vi "Read_From_File.vi"(8 "error in":errorcluster, 11 "user":i32) -> (0 "error out":errorcluster, 3 "Events":string)   [LabVIEW 2019]
panel:
  out "user":i32
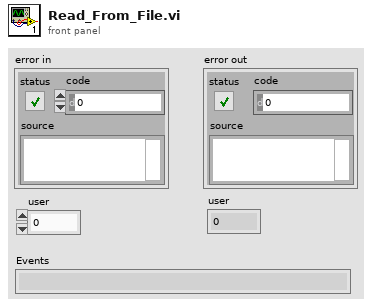
[diagram p1: front panel]
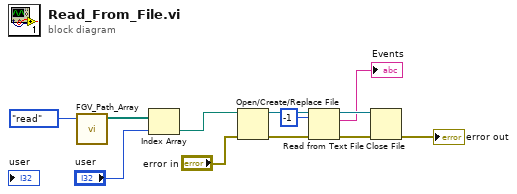
[diagram p0: block diagram]
diagram:
  n1 = call "FGV_Path_Array.vi"("Enum"=enum16{"read", "write"}."read" ("operation (0:open)")) -> ("path out"=w4:path[])  [unwired: 10 in]
  n2 = Index Array(array=w4, index="user") -> (element=w2:path)
  n3 = Open/Create/Replace File(file path (use dialog)=w2, error in="error in") -> (refnum out=w12:refnum<file>, error out=w9:errorcluster)  [unwired: 4 in, 1 out]
  n4 = Read from Text File(file (use dialog)=w12, count=-1, error in=w9) -> (refnum out=w11:refnum<file>, text=→"Events":string, error out=w6:errorcluster)  [unwired: 1 in, 1 out]
  n5 = Close File(refnum=w11, error in=w6) -> (error out=→"error out":errorcluster)  [unwired: 1 out]
